vi "ExSubSetupQ.vi"(2 "error in (no error)":errorcluster, 3 "Camera Handle":u32) -> (0 "error out":errorcluster, 1 "Camera Handle":u32)   [LabVIEW 2010]
panel:
  # "ExSubSetupCoolSnap:\nThis Sub VI sets up the skips, cleans, and shutter parameters.\nThis should be changed to suit the camera you are using."
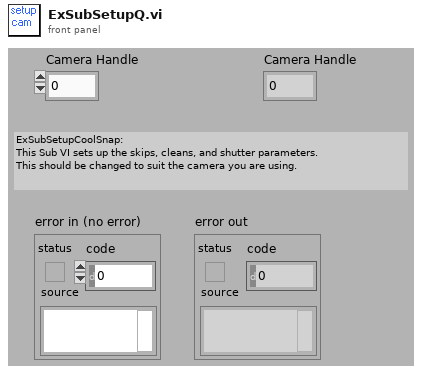
[diagram p1: front panel]
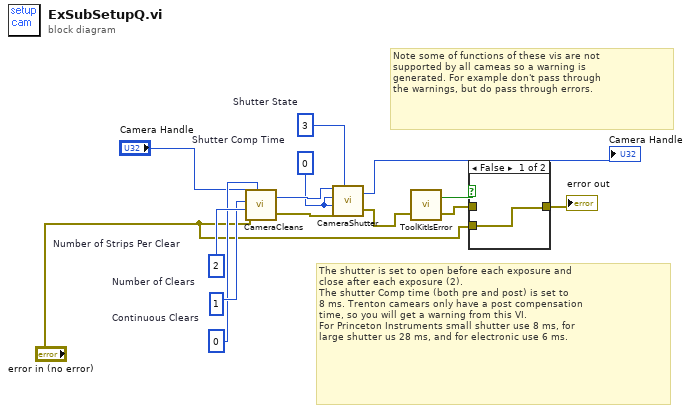
[diagram p0: block diagram]
diagram:
  w3 = u32 3  # Shutter State
  w4 = u32 0  # Shutter Comp Time
  w10 = u32 1  # Number of Clears
  w11 = u32 2  # Number of Strips Per Clear
  w9 = u32 0  # Continuous Clears
  # "Note some of functions of these vis are not \nsupported by all cameas so a warning is \ngenerated. For example don't pass through \nthe warnings, but do pass through errors."
  # "The shutter is set to open before each exposure and\nclose after each exposure (2).\nThe shutter Comp time (both pre and post) is set to \n8 ms. Trenton camears only have a post compensation \ntime, so you will get a warning from this VI.\nFor Princeton Instruments small shutter use 8 ms, for \nlarge shutter us 28 ms, and for electronic use 6 ms."
  n1 = call <userlib>:"CameraCleans.vi"("Camera Handle"="Camera Handle", "Number of Clears"=w10, "Number of Strips Per Clear"=w11, "error in"="error in (no error)", "Continuous Clears"=w9) -> ("Camera Handle"=w7:u32, "error out"=w8:errorcluster)
  n2 = call <userlib>:"CameraShutter.vi"("Camera Handle"=w7, "Shutter Comp Time: Pre Open"=w4, "Shutter Comp Time: Post Open"=w4, "error in"=w8, "Shutter State"=w3) -> ("Camera Handle"=→"Camera Handle":u32, "error out"=w6:errorcluster)
  n3 = call <userlib>:"ToolKitIsError.vi"("error in"=w6) -> ("error out"=w13:errorcluster, "Error Flag"=w14:bool)  [unwired: 1 in]
  n4 = case shown="False" w14 {
    tunnel: w13 -> [_ w16]
    tunnel: [w15 w16] -> w12
    tunnel: "error in (no error)" -> [w15 _]
    frame False {
    }
    frame True {
    }
  }
  "error out" <- w12
